vi "reflexe-audio-bis.vi"() -> (3 "reflexe (ms)":u32)   [LabVIEW 2025]
uses:
  <vilib>/numeric/Random Number (Range) U64.vi
  <vilib>/numeric/sub_Random U32.vi
panel:
  out "VOYANT":bool
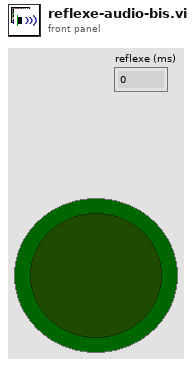
[diagram p1: front panel]
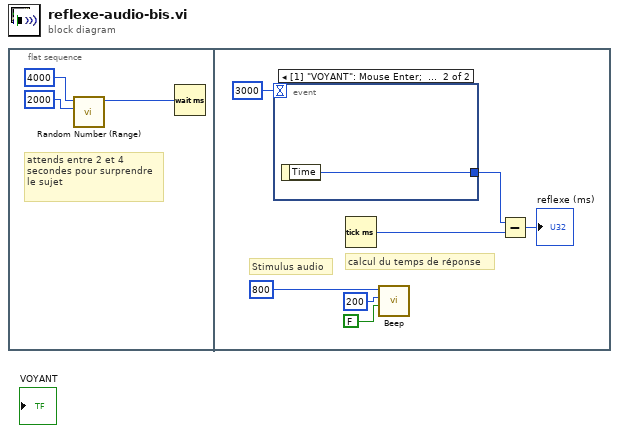
[diagram p0: block diagram]
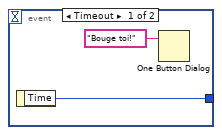
[diagram p2: hidden frame]
diagram:
  n1 = flat-sequence {
    frame #0 {
      # "attends entre 2 et 4 secondes pour surprendre le sujet"
      n2 = call-poly <vilib>:"Random Number (Range).vi"("lower bound (0)"=u64 2000, "upper bound (100)"=u64 4000) -> ("number"=w3:u64)  [unwired: 9 in]
      n3 = Wait (ms)(milliseconds to wait=w3) -> ()  [unwired: 1 out]
    }
    frame #1 {
      # "Stimulus audio"
      # "calcul du temps de réponse"
      n4 = event shown="[1] \"VOYANT\": Mouse Enter;  \"VOYANT\": Mouse Down" {
        selector: _ -> [_ _]
        dyn-events: _ -> [_ _]
        timeout: 3000 -> [_ _]
        tunnel: [w11 w13] -> w8
        event Timeout {
          n5 = event-data() -> ("Time"=w11:u32)  [unwired: 1 in]
          n6 = One Button Dialog(message="Bouge toi!") -> ()  [unwired: 1 in, 1 out]
        }
        event "VOYANT": Mouse Enter; "VOYANT": Mouse Down {
          n7 = event-data() -> ("Time"=w13:u32)  [unwired: 1 in]
        }
      }
      n8 = Tick Count (ms)() -> (millisecond timer value=w10:u32)
      n9 = call <vilib>:"Beep.vi"("use system alert? (T)"=FALSE, "duration (msec)"=u32 200, "frequency (Hz)"=u32 800) -> ()  [unwired: 9 in]
      n10 = Subtract(x=w8, y=w10) -> (x-y=→"reflexe (ms)":u32)
    }
  }
